vi "Do.vi"(8 "error in (no error)":errorcluster, 10 "Actor in":refnum<class "Actor.lvclass">, 11 "Set Item Configurations Msg":refnum<class "Set Item Configurations Msg.lvclass">) -> (0 "error out":errorcluster, 2 "Actor out":refnum<class "Actor.lvclass">)   [LabVIEW 2013, in "Create Test Channel Model.lvlib" / "Set Item Configurations Msg.lvclass"]
doc: "(<B>Filename</B>: Actor Framework.lvlib:Message.lvclass:Do.vi)\n\nDefines what a message does when it is received by an actor. Generally, a message instructs an actor to invoke one of its methods.\n\nBy default, this method does nothing. A child class must override it to define behavior. Create a child class by using the Actor Framework Message Maker dialog box."
uses:
  Set Item Configurations Msg.lvclass
  <vilib>/ActorFramework/Actor/Actor.lvclass
  Create Test Channel Model/Create Test Channel Model.lvclass
  Set Item Configurations Msg.lvclass/Set Item Configurations Msg.ctl
  Create Test Channel Model/Create Test Channel Model.lvclass/Create Test Channel Model.ctl
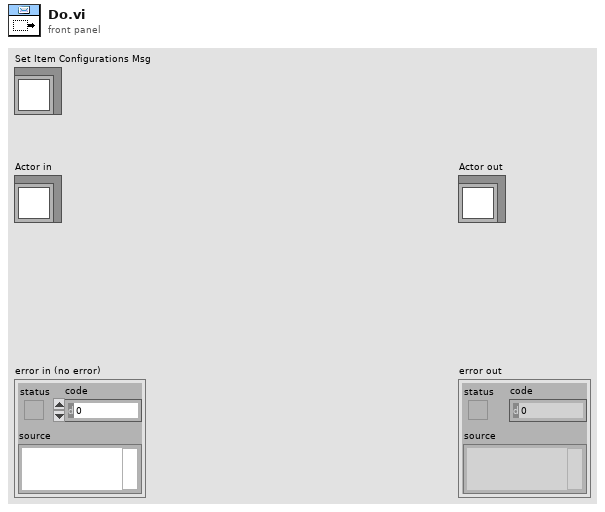
[diagram p1: front panel]
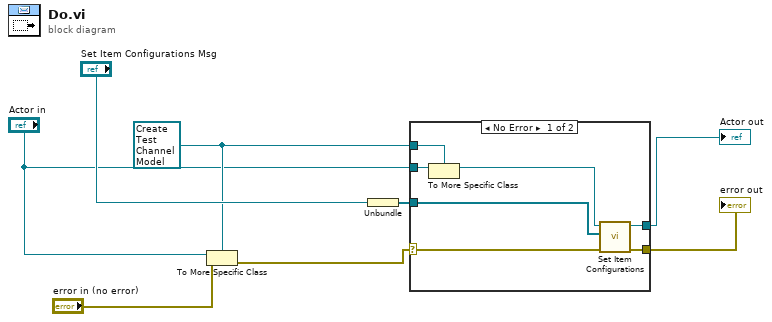
[diagram p0: block diagram]
diagram:
  w6 = refnum<class "Create Test Channel Model.lvclass"> refnum ("Create Test Channel Model.lvlib:Create Test Channel Model.lvclass")
  n1 = To More Specific Class(target class=w6, reference="Actor in", error in="error in (no error)") -> (error out=w4:errorcluster)  [unwired: 1 out]
  n2 = Unbundle("Set Item Configurations Msg") -> (w8:refnum<class "Item Configuration.lvclass">[])
  n3 = case shown="No Error" w4 {
    selector: w4 -> [w13 w17]
    tunnel: [w15 w17] -> w2
    tunnel: [w14 w16] -> w1
    tunnel: "Actor in" -> [w12 w16]
    tunnel: w6 -> [w11 _]
    tunnel: w8 -> [w9 _]
    frame No Error {
      n4 = To More Specific Class(target class=w11, reference=w12) -> (specific class reference=w10:refnum<class "Create Test Channel Model.lvclass">)  [unwired: 1 in, 1 out]
      n5 = call "Set Item Configurations.vi"("error in (no error)"=w13, "Item Configurations"=w9, "Create Test Channel Model in"=w10) -> ("error out"=w15:errorcluster, "Create Test Channel Model out"=w14:refnum<class "Create Test Channel Model.lvclass">)  [unwired: 7 in]
    }
    frame Error {
      # "If type check fails, pass the original object out again."
    }
  }
  "error out" <- w2
  "Actor out" <- w1
